vi "From Integer Tree Data.vi"(11 "Tree Data":refnum<class "Tree Data.lvclass">) -> (2 "Integer":i64)   [LabVIEW 2020, in "NI_VIAnCFGDataStructure.lvlib" / "Int.lvclass"]
doc: "Extract an Integer value from Tree Data type."
uses:
  <vilib>/addons/analyzer/VIAnCFGDataStructure/Data Types/Int/Int.lvclass
  <vilib>/addons/analyzer/VIAnCFGDataStructure/Tree Data/Tree Data.lvclass
  <vilib>/addons/analyzer/VIAnCFGDataStructure/Data Types/Int/Int.lvclass/Int.ctl
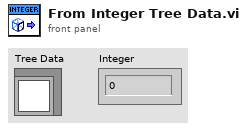
[diagram p1: front panel]
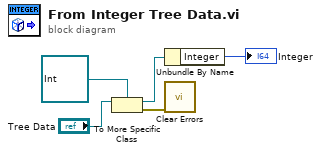
[diagram p0: block diagram]
diagram:
  n1 = To More Specific Class(target class=refnum<class "Int.lvclass"> refnum ("Int.lvclass"), reference="Tree Data") -> (specific class reference=w2:refnum<class "Int.lvclass">, error out=w4:errorcluster)  [unwired: 1 in]
  n2 = Unbundle By Name(w2) -> ("Integer"=→"Integer":i64)
  n3 = call <vilib>:"Clear Errors.vi"("error in (no error)"=w4) -> ()  [unwired: 5 in, 2 out]
